vi "Tree_Update Tree.vi"(4 "Close Items":bool, 6 "Disabled?":bool[](array[boolean]), 7 "Focus Item":string, 8 "error in":errorcluster, 9 "New Items":T1(array[cluster]), 10 "Show Changed":bool, 11 "TreeControl in":refnum<vi>) -> (0 "error out":errorcluster, 3 "TreeControl out":refnum<vi>)   [LabVIEW 2023]
doc: "Update tree with new items. If filtered, try to maintain position on change of show scripting/private."
uses:
  Libraries/Tree Handler/Tree Handlr.lvlib
panel:
  out "Array":string[](array[string])
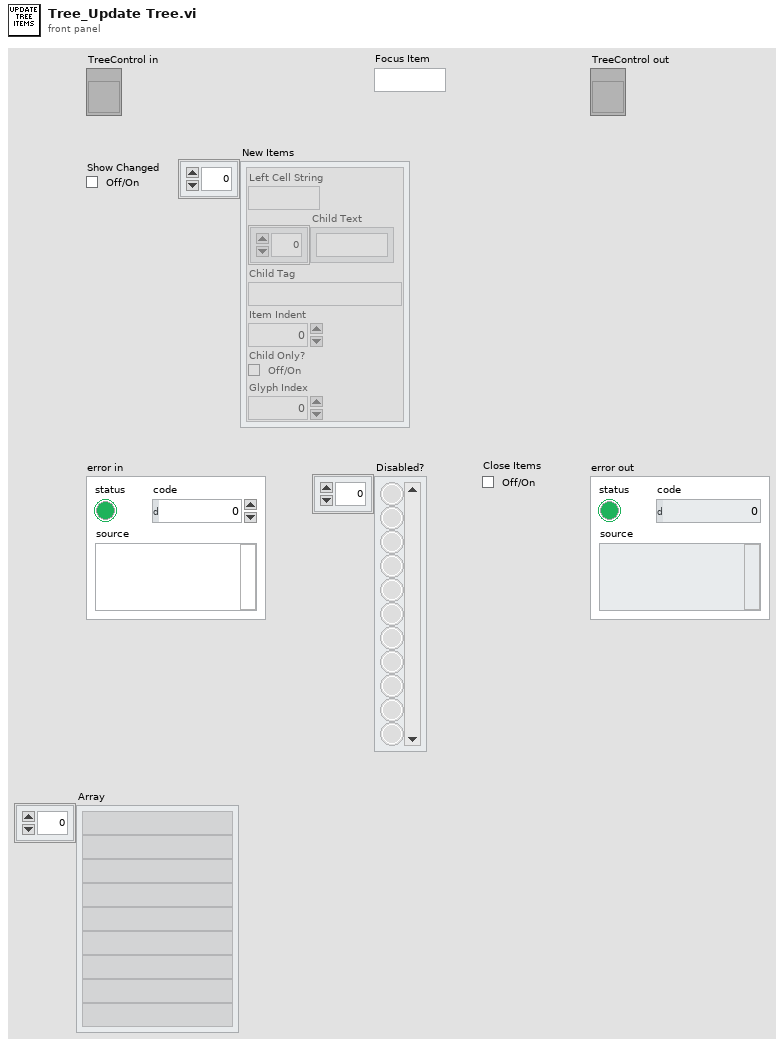
[diagram p1: front panel]
types:
  T1 = cluster{"Left Cell String":string, "Child Text":string[], "Child Tag":string, "Item Indent":i32, "Child Only?":bool, "Glyph Index":i32}[]
  T2 = typedef "LVNodeAndColumnTypeDef.ctl" = cluster{"Node":string, "Column":i32}
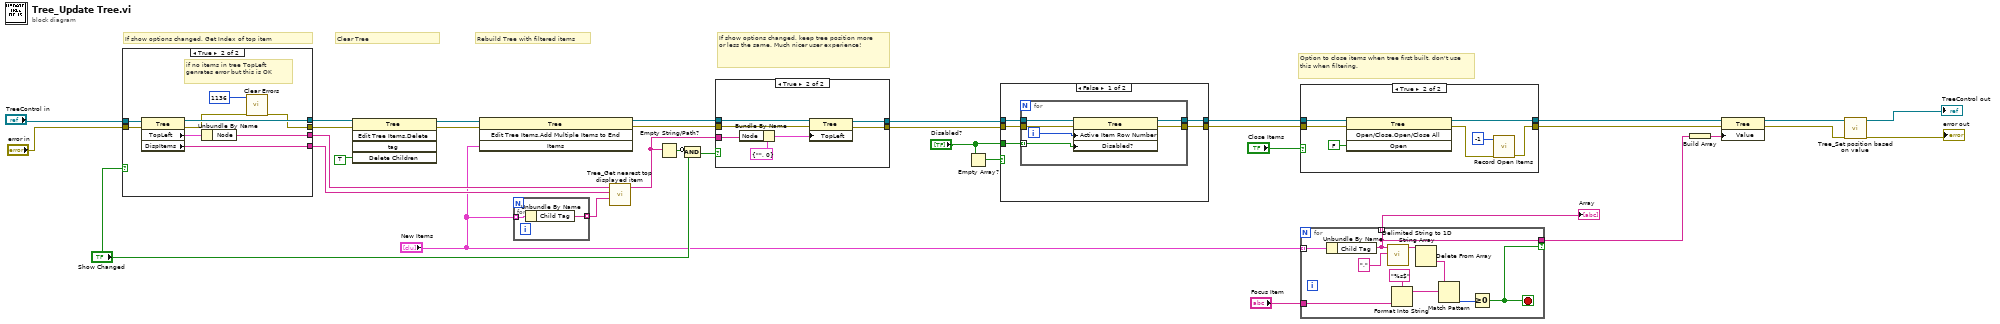
[diagram p0: block diagram]
diagram:
  # "Option to close items when tree first built, don't use this when filtering."
  # "If show options changed, keep tree position more or less the same. Much nicer user experience!"
  # "Rebuild Tree with filtered items"
  # "Clear Tree"
  # "If show options changed, Get Index of top item"
  n1 = case shown="True" "Show Changed" {
    tunnel: "TreeControl in" -> [w35 w45]
    tunnel: "error in" -> [w36 w44]
    tunnel: [w35 w43] -> w25
    tunnel: [w36 w38] -> w26
    tunnel: [_ w41] -> w30
    tunnel: [_ w40] -> w29
    frame False {
    }
    frame True {
      # "if no items in tree TopLeft genrates error but this is OK"
      n2 = property class="Tree"(reference=w45, error in=w44) -> (reference out=w43:refnum<vi>, error out=w39:errorcluster, "TopLeft"=w42:T2, "DispItems"=w40:string[])
      n3 = Unbundle By Name(w42) -> ("Node"=w41:string)
      n4 = call <vilib>:"Clear Errors.vi"("error in (no error)"=w39, "specific error code to clear (0: all)"=1136) -> ("error out"=w38:errorcluster)  [unwired: 4 in, 1 out]
    }
  }
  n5 = invoke class="Tree" method="Edit Tree Items.Delete"(reference=w25, error in=w26, "Delete Children"=TRUE ("Delete Children?")) -> (reference out=w21:refnum<vi>, error out=w22:errorcluster)  [unwired: 2 in, 3 out]
  n6 = invoke class="Tree" method="Edit Tree Items.Add Multiple Items to End"(reference=w21, error in=w22, "Items"="New Items") -> (reference out=w27:refnum<vi>, error out=w28:errorcluster)  [unwired: 1 in, 2 out]
  n7 = for {
    tunnel: "New Items" -> [w47] mode=indexing
    tunnel: [w46] -> w19 mode=indexing
    n8 = Unbundle By Name(w47) -> ("Child Tag"=w46:string)
  }
  n9 = call "Tree_Get nearest top displayed item.vi"("Retained Tags"=w19, "Original Tags"=w29, "Top Tag In"=w30) -> ("Top Tag Out"=w31:string)  [unwired: 8 in]
  n10 = Empty String/Path?(string/path=w31) -> (empty?=w32:bool)
  n11 = Compound Arithmetic op=AND(invert w32, "Show Changed") -> (w33:bool)
  n12 = case shown="True" w33 {
    tunnel: w27 -> [w49 w56]
    tunnel: [w49 w55] -> w17
    tunnel: w28 -> [w48 w54]
    tunnel: [w48 w50] -> w16
    tunnel: w31 -> [_ w51]
    frame False {
    }
    frame True {
      n13 = Bundle By Name(cluster=cluster{"Node":string, "Column":i32} {"Node"="", "Column"=0} ("Top Left Visible Cell"), "Node"=w51) -> (w53:cluster{"Node":string, "Column":i32})
      n14 = property class="Tree"(reference=w56, error in=w54, "TopLeft"=w53) -> (reference out=w55:refnum<vi>, error out=w50:errorcluster)
    }
  }
  n15 = Empty Array?(array="Disabled?") -> (empty?=w18:bool)
  n16 = case shown="False" w18 {
    tunnel: w17 -> [w61 w69]
    tunnel: [w60 w69] -> w14
    tunnel: w16 -> [w59 w68]
    tunnel: [w58 w68] -> w13
    tunnel: "Disabled?" -> [w57 _]
    frame False {
      n17 = for {
        tunnel: w61 -> [w67]
        tunnel: [w65] -> w60
        tunnel: w59 -> [w64]
        tunnel: [w63] -> w58
        tunnel: w57 -> [w62] mode=indexing
        i -> [w66]
        n18 = property class="Tree"(reference=w67, error in=w64, "Active Item Row Number"=w66, "Disabled?"=w62) -> (reference out=w65:refnum<vi>, error out=w63:errorcluster)
      }
    }
    frame True {
    }
  }
  n19 = case shown="True" "Close Items" {
    tunnel: w14 -> [w71 w78]
    tunnel: w13 -> [w70 w77]
    tunnel: [w71 w76] -> w5
    tunnel: [w70 w72] -> w4
    frame False {
    }
    frame True {
      n20 = invoke class="Tree" method="Open/Close.Open/Close All"(reference=w78, error in=w77, "Open"=FALSE ("Open?")) -> (reference out=w76:refnum<vi>, error out=w73:errorcluster)  [unwired: 1 in, 2 out]
      n21 = call "Record Open Items.vi"("error in"=w73, "Module ID"=-1) -> ("error out"=w72:errorcluster)  [unwired: 9 in]
    }
  }
  n22 = for {
    tunnel: "New Items" -> [w88] mode=indexing
    tunnel: "Focus Item" -> [w79]
    tunnel: [w85] -> w3 if=w82
    tunnel: [w85] -> w9 mode=indexing
    stop <- w82 stop-if-true
    n23 = Unbundle By Name(w88) -> ("Child Tag"=w85:string)
    n24 = call <vilib>:"Delimited String to 1D String Array.vi"("delimiter"=",", "delimited string"=w85) -> ("string array"=w86:string[])  [unwired: 9 in]
    n25 = Format Into String(format string="%s$", w79) -> (resulting string=w80:string)  [unwired: 2 in, 1 out]
    n26 = Delete From Array(array=w86) -> (deleted portion=w84:string)  [unwired: 2 in, 1 out]
    n27 = Match Pattern(string=w84, regular expression=w80) -> (offset past match=w83:i32)  [unwired: 1 in, 3 out]
    n28 = Greater Or Equal To 0?(x=w83) -> (x >= 0?=w82:bool)
  }
  "Array" <- w9
  n29 = Build Array(w3) -> (w2:string[])
  n30 = property class="Tree"(reference=w5, error in=w4, "Value"=w2) -> (reference out=w8:refnum<vi>, error out=w7:errorcluster)
  n31 = call "Tree_Set position based on value.vi"("error in (no error)"=w7, "Tree Ref"=w8) -> ("error out"=→"error out":errorcluster, "Tree Ref"=→"TreeControl out":refnum<vi>)  [unwired: 8 in]
